vi "Write View Channel info.vi"(8 "error in":errorcluster, 10 "channel info":T1, 11 "channel in":refnum<class "channel node.lvclass">) -> (0 "error out":errorcluster, 3 "channel out":refnum<class "channel node.lvclass">)   [LabVIEW 2013, in "channel node.lvclass"]
uses:
  channel node.lvclass
  ChannelDisplayInfo.ctl
  channel node.lvclass/channel node.ctl
  channel configuration/channel configuration.lvclass/channel configuration.ctl
  channel configuration/Write IO.vi
  channel configuration/Write sensor ID.vi
  channel configuration/Write channel name.vi
  channel configuration/Write description.vi
  channel configuration/channel configuration.lvclass
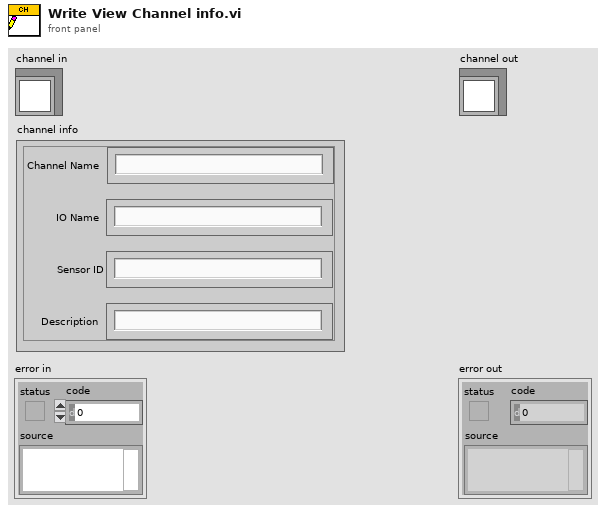
[diagram p1: front panel]
types:
  T1 = typedef "channel node.lvclass/ChannelDisplayInfo.ctl" = cluster{"IO Name":string, "Sensor ID":string, "Channel Name":string, "Description ":string}
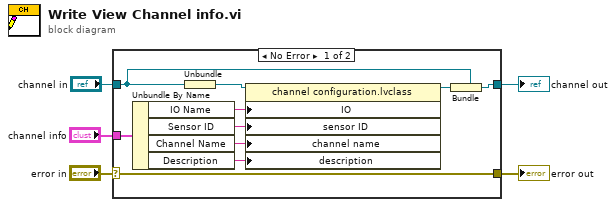
[diagram p0: block diagram]
diagram:
  n1 = case shown="No Error" "error in" {
    selector: "error in" -> [w15 w16]
    tunnel: [w15 w16] -> w4
    tunnel: [w12 w17] -> w2
    tunnel: "channel in" -> [w13 w17]
    tunnel: "channel info" -> [w14 _]
    frame No Error {
      n2 = Unbundle By Name(w14) -> ("IO Name"=w9:string, "Sensor ID"=w8:string, "Channel Name"=w7:string, "Description"=w6:string)
      n3 = Unbundle(w13) -> (w11:refnum<class "channel configuration.lvclass">)
      n4 = property class="channel configuration.lvclass"(reference=w11, "IO "=w9, "sensor ID"=w8, "channel name"=w7, "description"=w6) -> (reference out=w10:refnum<class "channel configuration.lvclass">)  [unwired: 1 in, 1 out]
      n5 = Bundle(cluster=w13, w10) -> (w12:refnum<class "channel node.lvclass">)
    }
    frame Error {
    }
  }
  "error out" <- w4
  "channel out" <- w2
